vi "Main_PXI_Test_3.vi"() -> ()   [LabVIEW 2018]
doc: "Main VI for the controls"
uses:
  Typedefs/StateDef_Enum.ctl
  <vilib>/Utility/error.llb/DialogType.ctl
  <vilib>/DAQmx/read.llb/DAQmx Read (Analog 1D DBL NChan 1Samp).vi
  <vilib>/DAQmx/write.llb/DAQmx Write (Analog DBL 1Chan 1Samp).vi
  <vilib>/DAQmx/create/channels.llb/DAQmx Create Channel (AO-Voltage-Basic).vi
  <vilib>/DAQmx/create/channels.llb/DAQmx Create Channel (AI-Voltage-Basic).vi
  <vilib>/DAQmx/configure/timing.llb/DAQmx Timing (Sample Clock).vi
  <vilib>/DAQmx/miscellaneous.llb/DAQmx Fill In Error Info.vi
  Components/Timing/Timing.lvlib
  <resource>/objmgr/daqmx.rc
panel:
  in  "System Stop Button":bool
  in  "Pause chart?":bool
  in  "Controller Params":enum32{"Page 1"}(tab)
  in  "Kp":dbl=1.0 min=0.0
  in  "Controller On?":bool
  out "Status":string
  in  "Loop Timing":enum32{"Ctrl.", "Ref. gen", "UI"}(tab)
  in  "Ctrl.\nLoop Rate (Hz)":dbl=25000.0 format="%#_4p"
  in  "ConvLateErrToWarning?":bool=TRUE
  in  "UI Loop rate (Hz)":dbl=1000.0 format="%#_6p"
  in  "Display Waveforms":enum32{"Controller Signals", "DSA "}(tab)
  out "Control Effort":dbl(graph)
  out "Waveform Chart":cluster{"Double":dbl, "Numeric":dbl}(graph)
  out "DSA Signals":cluster{"Double":dbl, "Double":dbl}(graph)
  # "Control Loop Timing"
  # "Ref.  Gen. Loop Timing"
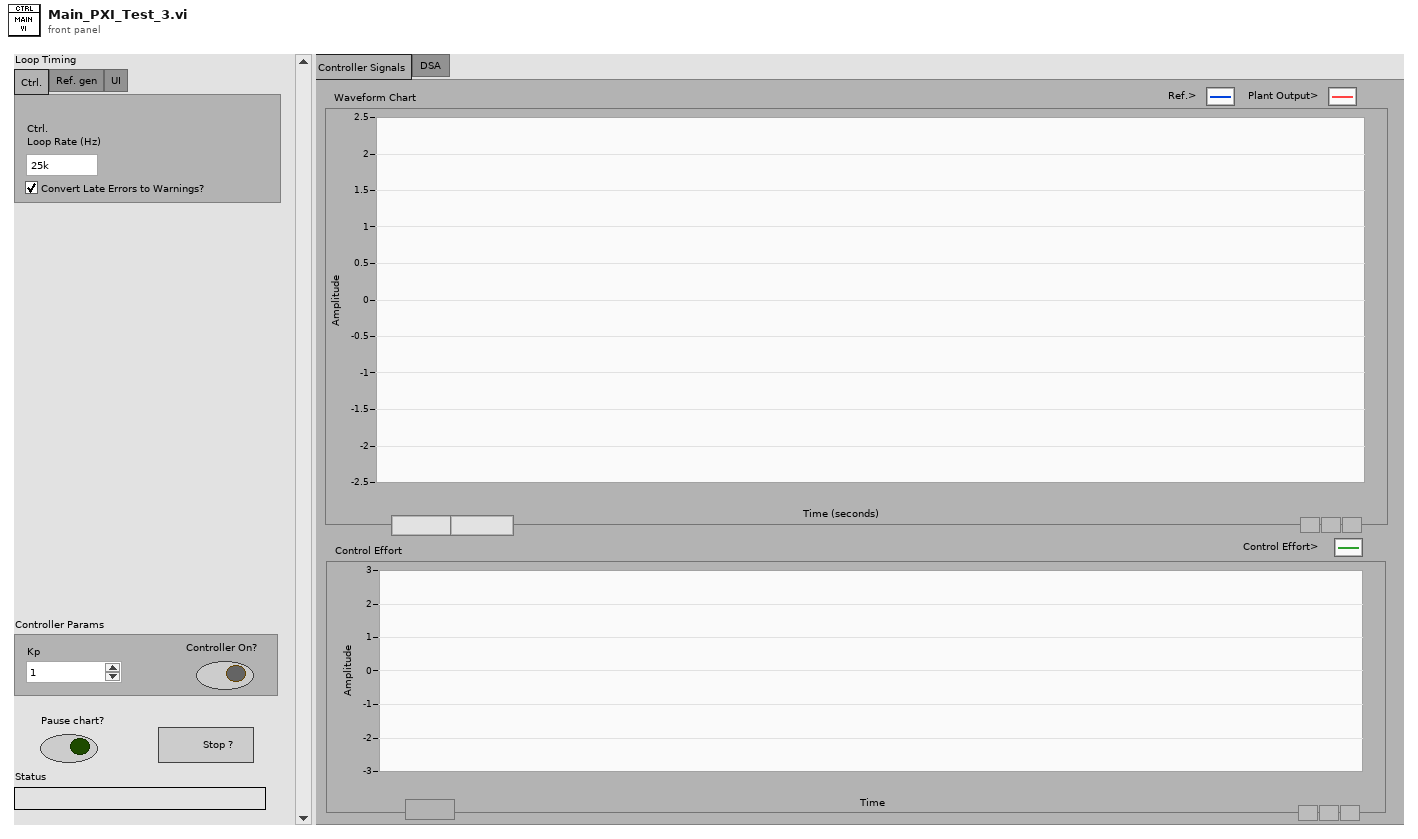
[diagram p1: front panel]
types:
  T1 = typedef "DialogType.ctl" = u16
  T2 = typedef "StateDef_Enum.ctl" = enum16{"Initialize", "Wait", "Shutdown"}
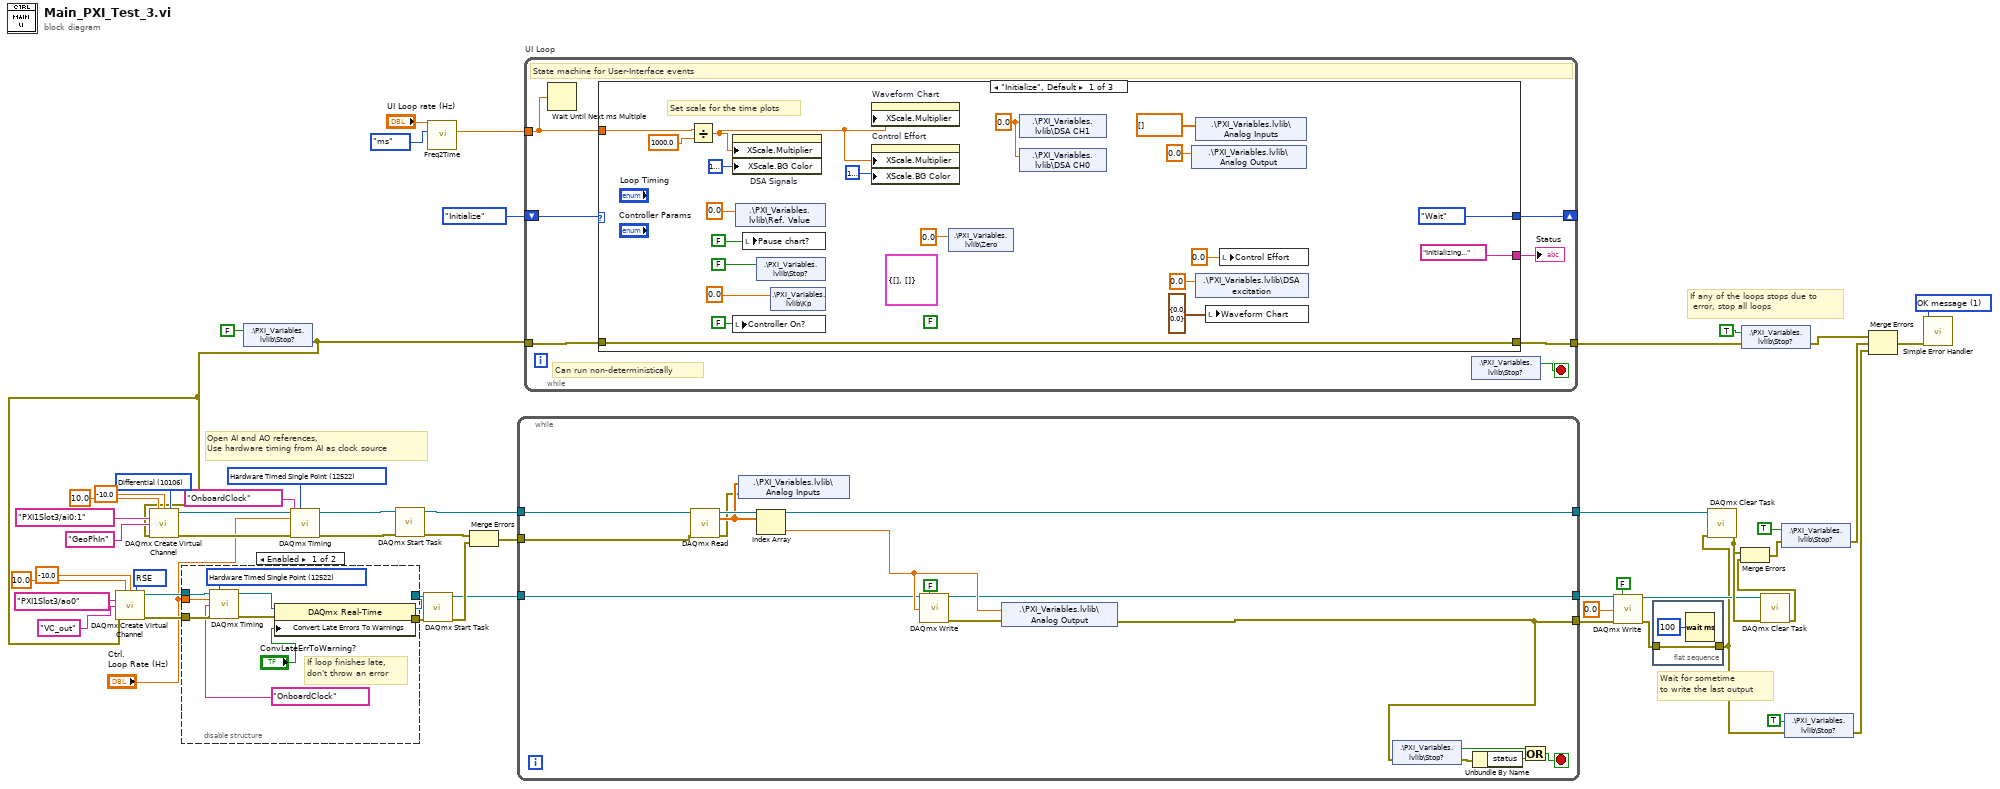
[diagram p0: block diagram]
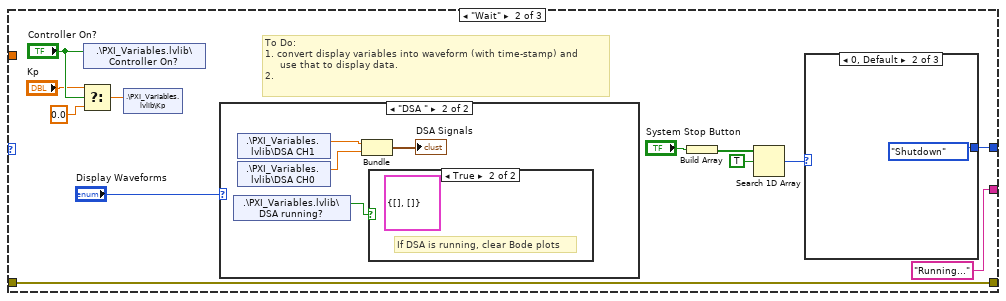
[diagram p3: hidden frame]
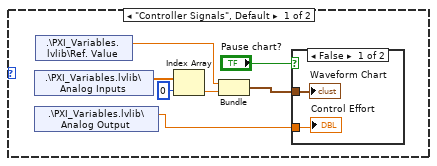
[diagram p4: hidden frame]
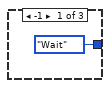
[diagram p7: hidden frame]
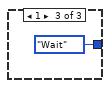
[diagram p8: hidden frame]
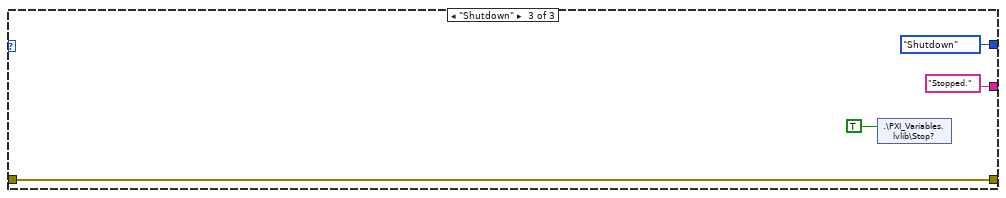
[diagram p9: hidden frame]
diagram:
  w23 = T1 1 items=["no dialog", "OK message", "continue or stop message", "OK message + warnings", "continue/stop + warnings"] ("type of dialog (OK msg:1)")
  w24 = 12522 items=["Finite Samples"=10178, "Continuous Samples"=10123, "Hardware Timed Single Point"=12522] ("sample mode")
  w36 = 10106 items=["Default"=-1, "RSE"=10083, "NRSE"=10078, "Differential"=10106, "Pseudodifferential"=12529] ("input terminal configuration")
  w39 = 10083 items=["Default"=-1, "RSE"=10083, "Differential"=10106, "Pseudodifferential"=12529] ("output terminal configuration")
  # "Wait for sometime \nto write the last output"
  # "Open AI and AO references,\nUse hardware timing from AI as clock source"
  # "If any of the loops stops due to\n error, stop all loops"
  n1 = shared-variable ".\\PXI_Variables.lvlib\\Stop?"(FALSE ("Stop?")) -> (error out=w22:errorcluster)  [unwired: 1 in]
  n2 = call-poly <vilib>:"DAQmx Create Virtual Channel.vi"("maximum value"=10.0, "minimum value"=-10.0, "output terminal configuration"=w39, "physical channels"=tag "PXI1Slot3/ao0", "name to assign"="VC_out", "error in"=w22) -> ("task out"=w15:refnum<k21>, "error out"=w14:errorcluster)  [unwired: 8 in]
  n3 = call-poly <vilib>:"DAQmx Create Virtual Channel.vi"("maximum value"=10.0, "minimum value"=-10.0, "input terminal configuration"=w36, "physical channels"=tag "PXI1Slot3/ai0:1", "name to assign"="GeoPhIn", "error in"=w22) -> ("task out"=w26:refnum<k21>, "error out"=w25:errorcluster)  [unwired: 8 in]
  n4 = disable-structure shown="Enabled" {
    disable-tunnel: w15 -> [w58 w64]
    disable-tunnel: w14 -> [w57 w63]
    disable-tunnel: "Ctrl.\nLoop Rate (Hz)" -> [w56 _]
    disable-tunnel: [w54 w63] -> w12
    disable-tunnel: [w53 w64] -> w10
    frame Enabled {
      w59 = 12522 items=["Finite Samples"=10178, "Continuous Samples"=10123, "Hardware Timed Single Point"=12522] ("sample mode")
      # "If loop finishes late,\ndon't throw an error"
      n5 = call-poly <vilib>:"DAQmx Timing.vi"("task/channels in"=w58, "sample mode"=w59, "rate"=w56, "source"=tag "OnboardClock", "error in"=w57) -> ("task out"=w61:refnum<k21>, "error out"=w60:errorcluster)  [unwired: 9 in]
      n6 = property class="DAQmx Real-Time"(reference=w61, error in=w60, "Convert Late Errors To Warnings"="ConvLateErrToWarning?") -> (reference out=w53:refnum<k21>, error out=w54:errorcluster)
    }
    frame Disabled {
    }
  }
  n7 = call-poly <vilib>:"DAQmx Timing.vi"("task/channels in"=w26, "sample mode"=w24, "rate"="Ctrl.\nLoop Rate (Hz)", "source"=tag "OnboardClock", "error in"=w25) -> ("task out"=w4:refnum<k21>, "error out"=w3:errorcluster)  [unwired: 9 in]
  n8 = call <vilib>:"DAQmx Start Task.vi"("task/channels in"=w4, "error in"=w3) -> ("task out"=w2:refnum<k21>, "error out"=w1:errorcluster)  [unwired: 12 in]
  n9 = call <vilib>:"DAQmx Start Task.vi"("task/channels in"=w10, "error in"=w12) -> ("task out"=w9:refnum<k21>, "error out"=w11:errorcluster)  [unwired: 12 in]
  n10 = call "Freq2Time.vi"("Int. Time Unit"=enum16{"sec", "us", "ms"}."ms", "Sample rate (Hz)"="UI Loop rate (Hz)") -> ("Int.  time [unit]"=w47:dbl)  [unwired: 7 in, 2 out]
  n11 = Merge Errors(w1, w11) -> (w7:errorcluster)
  n12 = while {
    tunnel: w2 -> [w79]
    tunnel: [w78] -> w27
    tunnel: w9 -> [w69]
    tunnel: [w66] -> w19
    tunnel: w7 -> [w68]
    tunnel: [w65] -> w6
    stop <- w73 stop-if-true
    n13 = call-poly <vilib>:"DAQmx Read.vi"("task/channels in"=w79, "error in"=w68) -> ("task out"=w78:refnum<k21>, "data"=w77:dbl[], "error out"=w72:errorcluster)  [unwired: 11 in]
    n14 = shared-variable ".\\PXI_Variables.lvlib\\Analog Inputs"(w77, error in=w72) -> ()  [unwired: 1 out]
    n15 = Index Array(array=w77) -> (element=w70:dbl)  [unwired: 1 in]
    n16 = call-poly <vilib>:"DAQmx Write.vi"("task/channels in"=w69, "auto start"=FALSE, "data"=w70) -> ("task out"=w66:refnum<k21>, "error out"=w67:errorcluster)  [unwired: 10 in, 1 out]
    n17 = shared-variable ".\\PXI_Variables.lvlib\\Analog Output"(w70, error in=w67) -> (error out=w65:errorcluster)
    n18 = shared-variable ".\\PXI_Variables.lvlib\\Stop?"(error in=w65) -> (w76:bool, error out=w75:errorcluster)
    n19 = Unbundle By Name(w75) -> ("status"=w74:bool)
    n20 = Or(x=w76, y=w74) -> (x .or. y?=w73:bool)
  }
  n21 = while "UI Loop" {
    shift-right: [w85] -> _
    shift-left: StateDef_Enum."Initialize" ("State defining Enum") -> [w86]
    tunnel: w22 -> [w84]
    tunnel: [w83] -> w46
    tunnel: w47 -> [w80]
    stop <- w81 stop-if-true
    # "Can run non-deterministically"
    # "State machine for User-Interface events"
    n22 = Wait Until Next ms Multiple(millisecond multiple=w80) -> ()  [unwired: 1 out]
    n23 = case shown="\"Initialize\", Default" w86 {
      tunnel: [StateDef_Enum."Wait" ("State defining Enum") w115 StateDef_Enum."Shutdown" ("State defining Enum")] -> w85
      tunnel: w84 -> [w103 w113 w138]
      tunnel: [w103 w113 w138] -> w83
      tunnel: ["Initializing..." ("Status") "Running..." ("Status") "Stopped." ("Status")] -> w82
      tunnel: w80 -> [w101 _ _]
      frame "Initialize", Default {
        w87 = 0.0 ("DSA CH1")
        (unwired) cluster{dbl[], dbl[]} {[], []} ("Magnitude Bode Plot")
        (unwired) FALSE ("DSA \nRunning?")
        # "Set scale for the time plots"
        n24 = Divide(x=w101, y=1000.0) -> (x/y=w95:dbl)
        n25 = property on="DSA Signals" class="WFChart (strict)"("XScale.Multiplier"=w95, "XScale.BG Color"=u32 16777216) -> ()  [unwired: 2 in, 2 out]
        n26 = local write "Controller On?"(FALSE ("Controller On?")) -> ()
        n27 = shared-variable ".\\PXI_Variables.lvlib\\Ref. Value"(0.0 ("Ref. Value")) -> ()  [unwired: 1 in, 1 out]
        n28 = local write "Pause chart?"(FALSE ("Pause chart?")) -> ()
        n29 = shared-variable ".\\PXI_Variables.lvlib\\Stop?"(FALSE ("Stop?")) -> ()  [unwired: 1 in, 1 out]
        n30 = shared-variable ".\\PXI_Variables.lvlib\\Kp"(0.0 ("Kp")) -> ()  [unwired: 1 in, 1 out]
        n31 = property on="Waveform Chart" class="WFChart (strict)"("XScale.Multiplier"=w95) -> ()  [unwired: 2 in, 2 out]
        n32 = property on="Control Effort" class="WFChart (strict)"("XScale.Multiplier"=w95, "XScale.BG Color"=u32 16777216) -> ()  [unwired: 2 in, 2 out]
        n33 = shared-variable ".\\PXI_Variables.lvlib\\Zero"(0.0 ("Zero")) -> ()  [unwired: 1 in, 1 out]
        n34 = shared-variable ".\\PXI_Variables.lvlib\\DSA CH1"(w87) -> ()  [unwired: 1 in, 1 out]
        n35 = shared-variable ".\\PXI_Variables.lvlib\\DSA CH0"(w87) -> ()  [unwired: 1 in, 1 out]
        n36 = shared-variable ".\\PXI_Variables.lvlib\\Analog Output"(0.0 ("Analog Output")) -> ()  [unwired: 1 in, 1 out]
        n37 = shared-variable ".\\PXI_Variables.lvlib\\Analog Inputs"(dbl[] [] ("Analog Inputs")) -> ()  [unwired: 1 in, 1 out]
        n38 = shared-variable ".\\PXI_Variables.lvlib\\DSA excitation"(0.0 ("DSA excitation")) -> ()  [unwired: 1 in, 1 out]
        n39 = local write "Waveform Chart"(cluster{"Double":dbl, "Numeric":dbl} {"Double"=0.0, "Numeric"=0.0} ("Waveform Chart")) -> ()
        n40 = local write "Control Effort"(0.0 ("Control Effort")) -> ()
      }
      frame "Wait" {
        # "To Do:\n1. convert display variables into waveform (with time-stamp) and\n     use that to display data.\n2."
        n41 = Select(t="Kp", s="Controller On?", f=0.0) -> (s? t:f=w111:dbl)
        n42 = shared-variable ".\\PXI_Variables.lvlib\\Controller On?"("Controller On?") -> ()  [unwired: 1 in, 1 out]
        n43 = shared-variable ".\\PXI_Variables.lvlib\\Kp"(w111) -> ()  [unwired: 1 in, 1 out]
        n44 = case shown="\"DSA \"" "Display Waveforms" {
          frame "Controller Signals", Default {
            n45 = shared-variable ".\\PXI_Variables.lvlib\\Analog Inputs"() -> (w125:dbl[])  [unwired: 1 in, 1 out]
            n46 = shared-variable ".\\PXI_Variables.lvlib\\Analog Output"() -> (w119:dbl)  [unwired: 1 in, 1 out]
            n47 = shared-variable ".\\PXI_Variables.lvlib\\Ref. Value"() -> (w122:dbl)  [unwired: 1 in, 1 out]
            n48 = Index Array(array=w125, index=0) -> (element=w124:dbl)
            n49 = Bundle("Double"=w122, "Numeric"=w124) -> (w120:cluster{"Double":dbl, "Numeric":dbl})  [unwired: 1 in]
            n50 = case shown="False" "Pause chart?" {
              tunnel: w120 -> [w127 _]
              tunnel: w119 -> [w126 _]
              frame False {
                "Waveform Chart" <- w127
                "Control Effort" <- w126
              }
              frame True {
              }
            }
          }
          frame "DSA " {
            n51 = shared-variable ".\\PXI_Variables.lvlib\\DSA running?"() -> (w128:bool)  [unwired: 1 in, 1 out]
            n52 = shared-variable ".\\PXI_Variables.lvlib\\DSA CH1"() -> (w130:dbl)  [unwired: 1 in, 1 out]
            n53 = shared-variable ".\\PXI_Variables.lvlib\\DSA CH0"() -> (w129:dbl)  [unwired: 1 in, 1 out]
            n54 = Bundle("Double"=w130, "Double"=w129) -> (→"DSA Signals":cluster{"Double":dbl, "Double":dbl})  [unwired: 1 in]
            n55 = case shown="True" w128 {
              frame False {
              }
              frame True {
                (unwired) cluster{dbl[], dbl[]} {[], []} ("Magnitude Bode Plot")
                # "If DSA is running, clear Bode plots"
              }
            }
          }
        }
        n56 = Build Array("System Stop Button") -> (w117:bool[])
        n57 = Search 1D Array(1D array=w117, element=TRUE) -> (index of element=w114:i32)  [unwired: 1 in]
        n58 = case shown="0, Default" w114 {
          tunnel: [StateDef_Enum."Wait" ("State defining Enum") StateDef_Enum."Shutdown" ("State defining Enum") StateDef_Enum."Wait" ("State defining Enum")] -> w115
          frame -1 {
          }
          frame 0, Default {
          }
          frame 1 {
          }
        }
      }
      frame "Shutdown" {
        n59 = shared-variable ".\\PXI_Variables.lvlib\\Stop?"(TRUE) -> ()  [unwired: 1 in, 1 out]
      }
    }
    "Status" <- w82
    n60 = shared-variable ".\\PXI_Variables.lvlib\\Stop?"() -> (w81:bool)  [unwired: 1 in, 1 out]
  }
  n61 = call-poly <vilib>:"DAQmx Write.vi"("task/channels in"=w19, "auto start"=FALSE, "data"=0.0, "error in"=w6) -> ("task out"=w16:refnum<k21>, "error out"=w17:errorcluster)  [unwired: 9 in, 1 out]
  n62 = flat-sequence {
    tunnel: [w140] -> w8
    tunnel: w17 -> [w140]
    frame #0 {
      n63 = Wait (ms)(milliseconds to wait=u32 100) -> ()  [unwired: 1 out]
    }
  }
  n64 = call <vilib>:"DAQmx Clear Task.vi"("task in"=w27, "error in"=w8) -> ("error out"=w20:errorcluster)  [unwired: 13 in]
  n65 = shared-variable ".\\PXI_Variables.lvlib\\Stop?"(TRUE ("Stop?"), error in=w46) -> (error out=w45:errorcluster)
  n66 = call <vilib>:"DAQmx Clear Task.vi"("task in"=w16, "error in"=w20) -> ("error out"=w30:errorcluster)  [unwired: 13 in]
  n67 = Merge Errors(w20, w30) -> (w31:errorcluster)
  n68 = shared-variable ".\\PXI_Variables.lvlib\\Stop?"(TRUE ("Stop?"), error in=w31) -> (error out=w28:errorcluster)
  n69 = shared-variable ".\\PXI_Variables.lvlib\\Stop?"(TRUE ("Stop?"), error in=w8) -> (error out=w29:errorcluster)
  n70 = Merge Errors(w45, w28, w29) -> (w51:errorcluster)
  n71 = call <vilib>:"Simple Error Handler.vi"("type of dialog (OK msg:1)"=w23, "error in (no error)"=w51) -> ()  [unwired: 3 in, 5 out]
